vi "Control File.vi"() -> (3 "Control File":string)   [LabVIEW 2015]
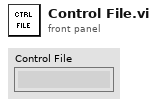
[diagram p1: front panel]
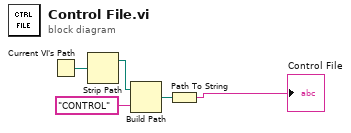
[diagram p0: block diagram]
diagram:
  n1 = Current VI's Path() -> (path=w3:path)
  n2 = Strip Path(path=w3) -> (stripped path=w2:path)  [unwired: 1 out]
  n3 = Build Path(base path=w2, name or relative path="CONTROL") -> (appended path=w5:path)
  n4 = Path To String(path=w5) -> (string=→"Control File":string)
